vi "RT Driver VI.vi"(7 "Operation":T1, 11 "Device Reference in":T2 format="%.0x") -> (0 "Error Code":i32)   [LabVIEW 2025, in "Runtime Configuration Support Example Engine.lvlib"]
uses:
  Runtime Configuration Support Example Engine.lvlib
  <vilib>/NI VeriStand/Custom Device API/Custom Device Item Ref.ctl
  <vilib>/NI VeriStand/Custom Device API/Hardware Interface Driver VI Operation.ctl
  <vilib>/NI VeriStand/Custom Device API/Custom Device Channel Type.ctl
  HW Operations.ctl
  Shared/Compiled.Settings.ctl
  <vilib>/NI VeriStand/Custom Device API/Data Access Type.ctl
  Command Loop.vi
  <vilib>/NI VeriStand/Custom Device API/Global Data Refs.vi
  <vilib>/NI VeriStand/Custom Device API/Custom Device API.lvlib
  Shared/Runtime Configuration Support Example Shared.lvlib
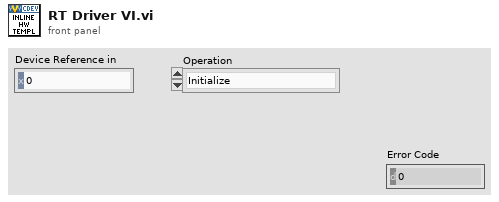
[diagram p1: front panel]
types:
  T1 = typedef "Custom Device API.lvlib/Hardware Interface Driver VI Operation.ctl" = enum16{"Initialize", "Start", "Read Data from HW", "Write Data to HW", "Close"}
  T2 = typedef "Custom Device API.lvlib/Custom Device Item Ref.ctl" = u64
  T3 = typedef "Runtime Configuration Support Example Shared.lvlib/Compiled.Settings.ctl" = cluster{"Name":string, "Inport SignalIDs":i32[], "Outport SignalIDs":i32[], "Inport Channel refs":T2[], "Outport Channel refs":T2[], "Inport Values":dbl[], "Outport Values":dbl[], "Device Error":errorcluster, "Dynamic Config Status":bool, "Response Ref":refnum<queue>}
  T4 = cluster{"Compiled Info":refnum<queue>, "Set HW Val Ref":refnum<queue>, "Get HW Val Ref":refnum<queue>}
  T5 = cluster{"SignalIDs In":i32[], "SignalIDs Out":i32[], "Response Ref":refnum<queue>}
  T6 = cluster{"SignalIDs":i32[], "Values":i32[], "Response Ref":refnum<queue>}
  T7 = typedef "HW Operations.ctl" = enum16{"Initialize", "Set In Val", "Get In Val", "Set Block", "Set Out Val", "Get Out Val", "Get In Array", "Get Out Array"}
  T8 = typedef "Custom Device API.lvlib/Custom Device Channel Type.ctl" = enum16{"Input", "Output"}
  T9 = typedef "Custom Device API.lvlib/Data Access Type.ctl" = enum16{"Read", "Write"}
  T10 = typedef "Custom Device API.lvlib/Data Reference.ctl" = i32
  T11 = cluster{bool, "Inport Values":dbl[], "Outport Values":dbl[], "error IO":errorcluster}
  T12 = cluster{"In Indices":i32[], "Out Indices":i32[], "Response Ref":refnum<queue>}
  T13 = cluster{"Indices":i32[], "Values":i32[], "Response Ref":refnum<queue>}
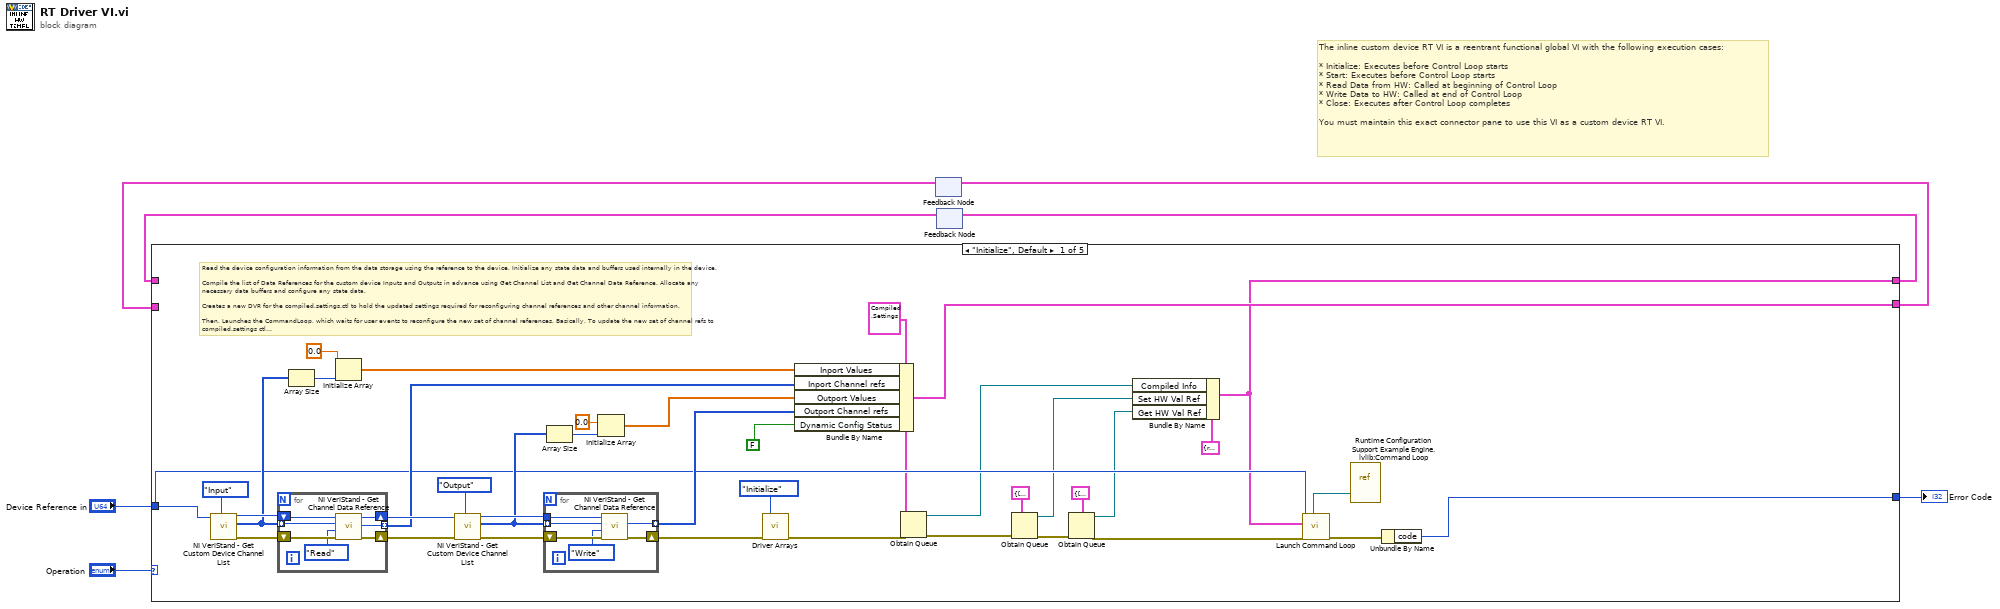
[diagram p0: block diagram]
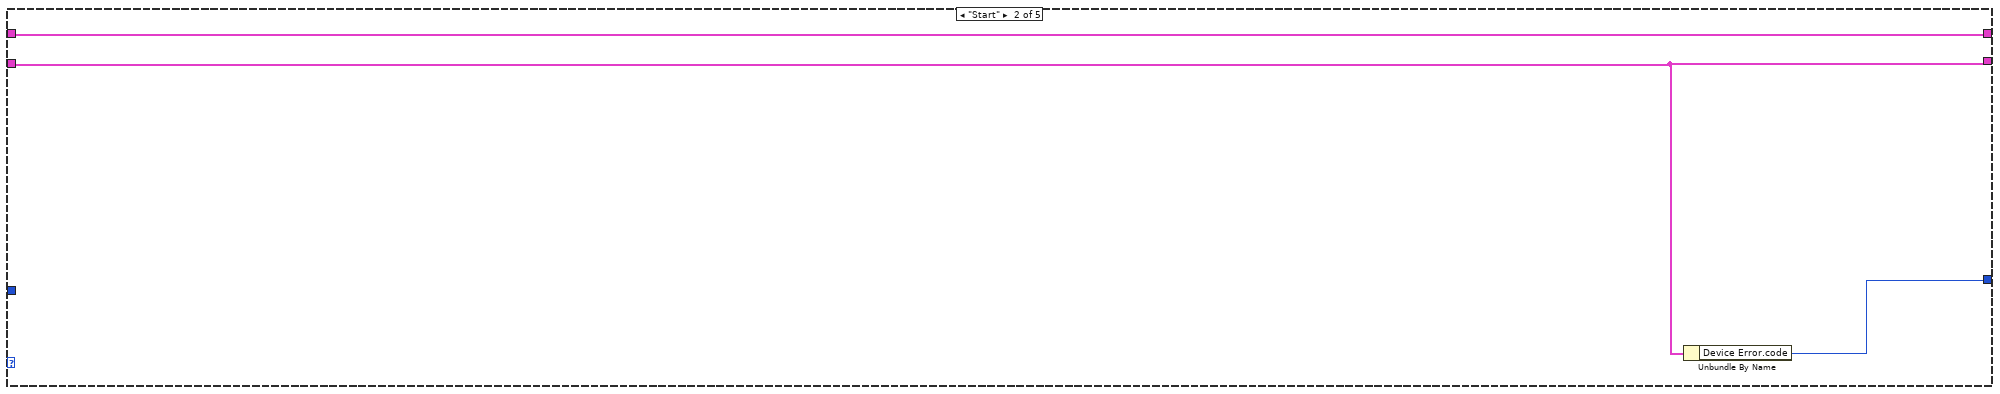
[diagram p2: hidden frame]
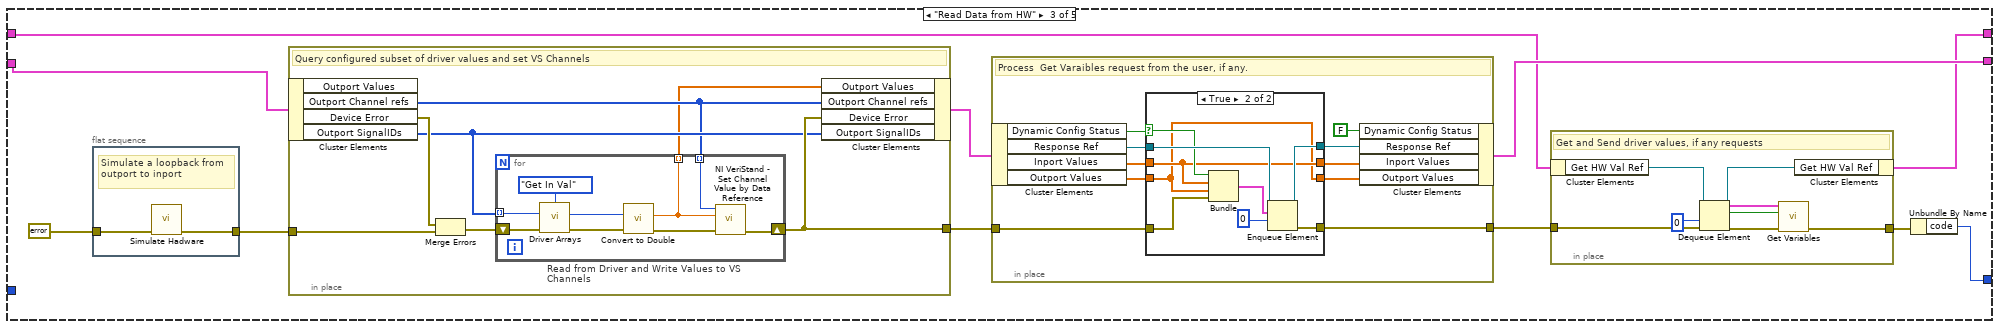
[diagram p3: hidden frame]
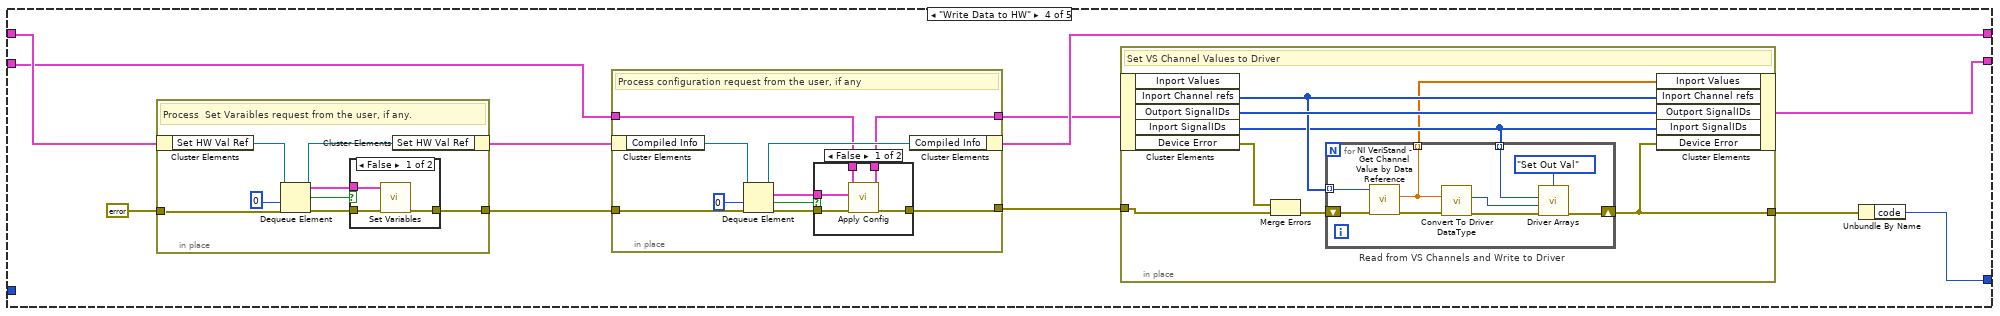
[diagram p5: hidden frame]
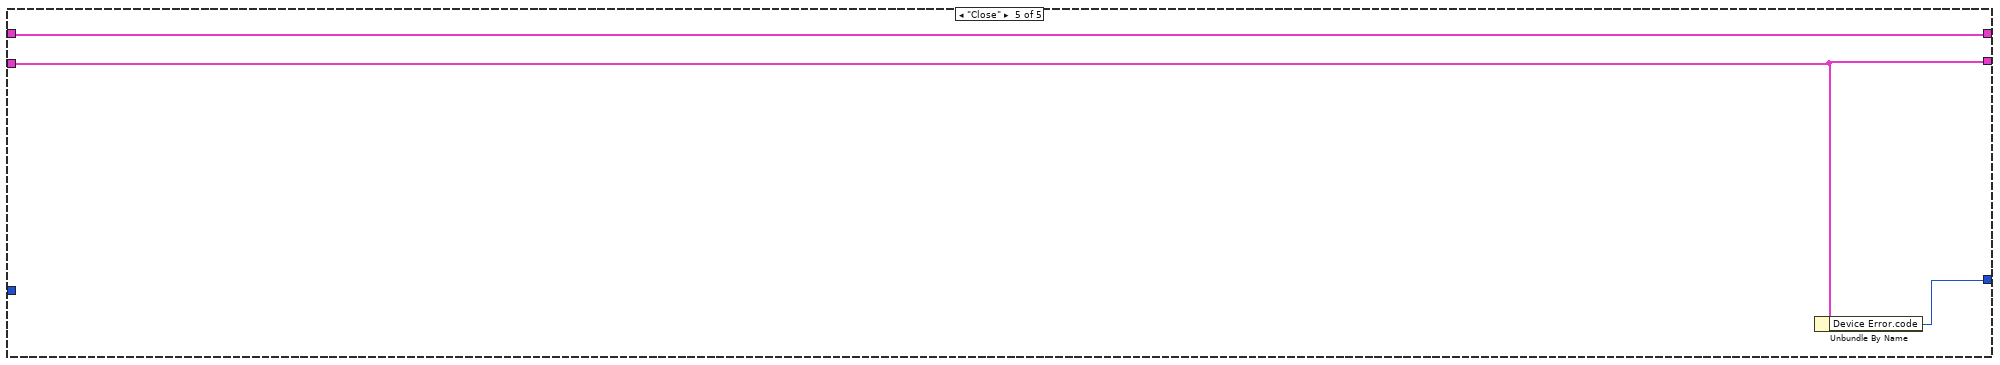
[diagram p8: hidden frame]
diagram:
  # "The inline custom device RT VI is a reentrant functional global VI with the following execution cases:\n\n* Initialize: Executes before Control Loop starts\n* Start: Executes before Control Loop starts\n* Read Data from HW: Called at beginning of Control Loop\n* Write Data to HW: Called at end of Control Loop\n* Close: Executes after Control Loop completes\n\nYou must maintain this exact connector pane to use this VI as a custom device RT VI."
  n1 = feedback #1() -> (w5:T3)  [unwired: 1 out]
  n2 = feedback #2() -> (w1:T4)  [unwired: 1 in]
  n3 = case shown="\"Initialize\", Default" "Operation" {
    tunnel: [w20 w60 w64 w121 w179] -> w6
    tunnel: w5 -> [_ w60 w66 w125 w179]
    tunnel: "Device Reference in" -> [w16 _ _ _ _]
    tunnel: [w33 w61 w67 w127 w180] -> w3
    tunnel: [w8 w59 w62 w123 w178] -> w2
    tunnel: w1 -> [_ w59 w63 w126 w178]
    frame "Initialize", Default {
      w15 = T3 {"Name"="", "Inport SignalIDs"=[], "Outport SignalIDs"=[], "Inport Channel refs"=[], "Outport Channel refs"=[], "Inport Values"=[], "Outport Values"=[], "Device Error"={"status"=FALSE, "code"=0, "source"=""}, "Dynamic Config Status"=FALSE, "Response Ref"=refnum} ("Compiled.Settings")
      # "Read the device configuration information from the data storage using the reference to the device. Initialize any state data and buffers used internally in the device.\n\nCompile the list of Data References for the custom device Inputs and Outputs in advance using Get Channel List and Get Channel Data Reference. Allocate any necessary data buffers and configure any state data.\n\nCreates a new DVR for the compiled.settings.ctl to hold the updated settings required for reconfiguring channel references and other channel information.\n\nThen, Launches the CommandLoop, which waits for user events to reconfigure the new set of channel references. Basically, To update the new set of channel refs to compiled.settings ctl\n\nYou can't read or write channel values in this case."
      n4 = call <vilib>:"NI VeriStand - Get Custom Device Channel List.vi"("Channel Type"=Custom_Device_Channel_Type."Input", "Device Ref in"=w16) -> ("error out"=w45:errorcluster, "Specified Channel Ref List"=w31:T2[], "Device Ref out"=w32:T2)  [unwired: 1 in, 6 out]
      n5 = for {
        shift-right: [w47] -> w28
        shift-left: w32 -> [w50]
        tunnel: w31 -> [w49] mode=indexing
        shift-right: [w51] -> w43
        shift-left: w45 -> [w52]
        tunnel: [w46] -> w19 mode=indexing
        n6 = call <vilib>:"NI VeriStand - Get Channel Data Reference.vi"("error in (no error)"=w52, "Access"=Data_Access_Type."Read", "Channel Ref in"=w49, "Device Ref in"=w50) -> ("error out"=w51:errorcluster, "Channel Data Reference"=w46:T10, "Device Ref out"=w47:T2)  [unwired: 5 out]
      }
      n7 = Array Size(array=w31) -> (size(s)=w36:i32)
      n8 = Initialize Array(0.0 ("element"), w36) -> (w22:dbl[])
      n9 = call <vilib>:"NI VeriStand - Get Custom Device Channel List.vi"("Channel Type"=Custom_Device_Channel_Type."Output", "error in (no error)"=w43, "Device Ref in"=w28) -> ("error out"=w44:errorcluster, "Specified Channel Ref List"=w25:T2[], "Device Ref out"=w30:T2)  [unwired: 6 out]
      n10 = for {
        tunnel: w25 -> [w55] mode=indexing
        shift-right: [w57] -> w41
        shift-left: w44 -> [w58]
        tunnel: [w53] -> w21 mode=indexing
        tunnel: w30 -> [w56]
        n11 = call <vilib>:"NI VeriStand - Get Channel Data Reference.vi"("error in (no error)"=w58, "Access"=Data_Access_Type."Write", "Channel Ref in"=w55, "Device Ref in"=w56) -> ("error out"=w57:errorcluster, "Channel Data Reference"=w53:T10)  [unwired: 6 out]
      }
      n12 = Array Size(array=w25) -> (size(s)=w26:i32)
      n13 = Initialize Array(0.0 ("element"), w26) -> (w18:dbl[])
      n14 = call "Driver Arrays.vi"("error in"=w41, "Curr Operation"=HW_Operations."Initialize") -> ("error out"=w40:errorcluster)  [unwired: 6 in, 3 out]
      n15 = Bundle By Name(cluster=w15, "Inport Values"=w22, "Inport Channel refs"=w19, "Outport Values"=w18, "Outport Channel refs"=w21, "Dynamic Config Status"=FALSE) -> (w20:T3)
      n16 = Obtain Queue(element data type=w15, error in (no error)=w40) -> (queue out=w9:refnum<queue>, error out=w39:errorcluster)  [unwired: 3 in, 1 out]
      n17 = Obtain Queue(element data type=T6 {"SignalIDs"=[], "Values"=[], "Response Ref"=refnum}, error in (no error)=w39) -> (queue out=w12:refnum<queue>, error out=w38:errorcluster)  [unwired: 3 in, 1 out]
      n18 = Obtain Queue(element data type=T5 {"SignalIDs In"=[], "SignalIDs Out"=[], "Response Ref"=refnum}, error in (no error)=w38) -> (queue out=w11:refnum<queue>, error out=w37:errorcluster)  [unwired: 3 in, 1 out]
      n19 = Bundle By Name(cluster=T4 {"Compiled Info"=refnum, "Set HW Val Ref"=refnum, "Get HW Val Ref"=refnum}, "Compiled Info"=w9, "Set HW Val Ref"=w12, "Get HW Val Ref"=w11) -> (w8:T4)
      n20 = vi-ref "Runtime Configuration Support Example Engine.lvlib:Command Loop.vi"() -> (w24:refnum<vi>)
      n21 = call "Launch Command Loop.vi"("VI Refnum"=w24, "error in"=w37, "Queue Refs"=w8, "Device Reference in"=w16) -> ("error out"=w42:errorcluster)  [unwired: 7 in]
      n22 = Unbundle By Name(w42) -> ("code"=w33:i32)
    }
    frame "Start" {
      n23 = Unbundle By Name(w60) -> ("Device Error.code"=w61:i32)
    }
    frame "Read Data from HW" {
      n24 = flat-sequence "Simulate HW" {
        tunnel: [w120] -> w71
        tunnel: errorcluster {"status"=FALSE, "code"=0, "source"=""} ("error in (no error)") -> [w119]
        frame #0 {
          # "Simulate a loopback from outport to inport"
          n25 = call "Simulate Hadware.vi"("error in"=w119) -> ("error out"=w120:errorcluster)  [unwired: 10 in]
        }
      }
      n26 = in-place "In Place Element Structure" {
        in-place-border: w71 -> [w108]
        in-place-border: [w106] -> w68
        # "Query configured subset of driver values and set VS Channels"
        n27 = in-place-cluster #3(w66) -> ("Outport Channel refs"=w104:T2[], "Device Error"=w109:errorcluster, "Outport SignalIDs"=w105:i32[])  [unwired: 1 out]
        n28 = Merge Errors(w109, w108) -> (w107:errorcluster)
        n29 = for "Read from Driver and Write Values to VS Channels" {
          shift-right: [w116] -> w106
          shift-left: w107 -> [w118]
          tunnel: w105 -> [w114] mode=indexing
          tunnel: w104 -> [w111] mode=indexing
          tunnel: [w110] -> w103 mode=indexing
          n30 = call "Driver Arrays.vi"("error in"=w118, "Index"=w114, "Curr Operation"=HW_Operations."Get In Val") -> ("error out"=w117:errorcluster, "Value"=w112:i32)  [unwired: 5 in, 2 out]
          n31 = call "Convert to Double.vi"("error in"=w117, "In"=w112) -> ("error out"=w115:errorcluster, "Out"=w110:dbl)  [unwired: 8 in]
          n32 = call <vilib>:"NI VeriStand - Set Channel Value by Data Reference.vi"("error in (no error)"=w115, "Value"=w110, "Data Reference in"=w111) -> ("error out"=w116:errorcluster)  [unwired: 8 out]
        }
        n33 = in-place-cluster #3("Outport Values"=w103, "Outport Channel refs"=w104, "Device Error"=w106, "Outport SignalIDs"=w105) -> (w65:T3)
      }
      n34 = in-place {
        in-place-border: [w90] -> w70
        in-place-border: w68 -> [w89]
        # "Process  Get Varaibles request from the user, if any."
        n35 = in-place-cluster #4(w65) -> ("Dynamic Config Status"=w86:bool, "Response Ref"=w88:refnum<queue>, "Inport Values"=w84:dbl[], "Outport Values"=w83:dbl[])
        n36 = case shown="True" w86 {
          selector: w86 -> [_ w97]
          tunnel: [_ w102] -> w90
          tunnel: w88 -> [w93 w100]
          tunnel: [w93 w98] -> w87
          tunnel: w84 -> [w92 w96]
          tunnel: w83 -> [w91 w95]
          tunnel: [w92 w96] -> w82
          tunnel: [w91 w95] -> w81
          tunnel: w89 -> [_ w101]
          frame False {
          }
          frame True {
            n37 = Bundle(w97, "Inport Values"=w96, "Outport Values"=w95, "error IO"=w101) -> (w94:T11)  [unwired: 1 in]
            n38 = Enqueue Element(queue=w100, element=w94, timeout in ms (-1)=0) -> (queue out=w98:refnum<queue>, error out=w102:errorcluster)  [unwired: 1 in, 1 out]
          }
        }
        n39 = in-place-cluster #4("Dynamic Config Status"=FALSE, "Response Ref"=w87, "Inport Values"=w82, "Outport Values"=w81) -> (w64:T3)
      }
      n40 = in-place {
        in-place-border: [w80] -> w69
        in-place-border: w70 -> [w79]
        # "Get and Send driver values, if any requests"
        n41 = in-place-cluster #5(w63) -> ("Get HW Val Ref"=w74:refnum<queue>)
        n42 = Dequeue Element(queue=w74, timeout in ms (-1)=0, error in (no error)=w79) -> (queue out=w76:refnum<queue>, element=w75:T12, timed out?=w77:bool, error out=w78:errorcluster)
        n43 = call "Get Variables.vi"("error in"=w78, "timed out?"=w77, "Data"=w75) -> ("error out"=w80:errorcluster)  [unwired: 8 in]
        n44 = in-place-cluster #5("Get HW Val Ref"=w76) -> (w62:T4)
      }
      n45 = Unbundle By Name(w69) -> ("code"=w67:i32)
    }
    frame "Write Data to HW" {
      n46 = in-place "In Place Element Structure" {
        in-place-border: [w172] -> w130
        in-place-border: errorcluster {"status"=FALSE, "code"=0, "source"=""} ("error in (no error)") -> [w171]
        # "Process  Set Varaibles request from the user, if any."
        n47 = in-place-cluster #6(w126) -> ("Set HW Val Ref"=w168:refnum<queue>)
        n48 = Dequeue Element(queue=w168, timeout in ms (-1)=0, error in (no error)=w171) -> (queue out=w167:refnum<queue>, element=w170:T13, timed out?=w166:bool, error out=w173:errorcluster)
        n49 = case shown="False" w166 {
          tunnel: w173 -> [w176 w177]
          tunnel: w170 -> [w174 _]
          tunnel: [w175 w177] -> w172
          frame False {
            n50 = call "Set Variables.vi"("error in (no error)"=w176, "Data"=w174) -> ("error out"=w175:errorcluster)  [unwired: 9 in]
          }
          frame True {
          }
        }
        n51 = in-place-cluster #6("Set HW Val Ref"=w167) -> (w124:T4)
      }
      n52 = in-place {
        in-place-border: w125 -> [w152]
        in-place-border: [w150] -> w122
        in-place-border: w130 -> [w158]
        in-place-border: [w156] -> w129
        # "Process configuration request from the user, if any"
        n53 = in-place-cluster #7(w124) -> ("Compiled Info"=w154:refnum<queue>)
        n54 = Dequeue Element(queue=w154, timeout in ms (-1)=0, error in (no error)=w158) -> (queue out=w153:refnum<queue>, element=w151:T3, timed out?=w149:bool, error out=w157:errorcluster)
        n55 = case shown="False" w149 {
          tunnel: w157 -> [w163 w165]
          tunnel: [w162 w165] -> w156
          tunnel: w152 -> [w161 w164]
          tunnel: w151 -> [w160 _]
          tunnel: [w159 w164] -> w150
          frame False {
            n56 = call "Apply Config.vi"("error in"=w163, "Data"=w160, "Compiled.Settings in"=w161) -> ("error out"=w162:errorcluster, "Compiled.Settings out"=w159:T3)  [unwired: 7 in]
          }
          frame True {
          }
        }
        n57 = in-place-cluster #7("Compiled Info"=w153) -> (w123:T4)
      }
      n58 = in-place {
        in-place-border: w129 -> [w138]
        in-place-border: [w136] -> w128
        # "Set VS Channel Values to Driver"
        n59 = in-place-cluster #8(w122) -> ("Inport Channel refs"=w134:T2[], "Outport SignalIDs"=w135:i32[], "Inport SignalIDs"=w133:i32[], "Device Error"=w139:errorcluster)  [unwired: 1 out]
        n60 = Merge Errors(w139, w138) -> (w137:errorcluster)
        n61 = for "Read from VS Channels and Write to Driver" {
          shift-right: [w145] -> w136
          shift-left: w137 -> [w148]
          tunnel: w134 -> [w144] mode=indexing
          tunnel: w133 -> [w141] mode=indexing
          tunnel: [w140] -> w132 mode=indexing
          n62 = call <vilib>:"NI VeriStand - Get Channel Value by Data Reference.vi"("error in (no error)"=w148, "Data Reference in"=w144) -> ("error out"=w147:errorcluster, "Value"=w140:dbl)  [unwired: 8 in]
          n63 = call "Convert To Driver DataType.vi"("error in"=w147, "In"=w140) -> ("error out"=w146:errorcluster, "Out"=w142:i32)  [unwired: 8 in]
          n64 = call "Driver Arrays.vi"("error in"=w146, "Value"=w142, "Index"=w141, "Curr Operation"=HW_Operations."Set Out Val") -> ("error out"=w145:errorcluster)  [unwired: 4 in, 3 out]
        }
        n65 = in-place-cluster #8("Inport Values"=w132, "Inport Channel refs"=w134, "Outport SignalIDs"=w135, "Inport SignalIDs"=w133, "Device Error"=w136) -> (w121:T3)
      }
      n66 = Unbundle By Name(w128) -> ("code"=w127:i32)
    }
    frame "Close" {
      n67 = Unbundle By Name(w179) -> ("Device Error.code"=w180:i32)
    }
  }
  "Error Code" <- w3
  n68 = feedback-in #1(w6) -> ()
  n69 = feedback-in #2(w2) -> ()
